vi "generate_plot.vi"(6 "High Voltage":sgl=2.0, 7 "Sens":dbl=12100000000000.0, 8 "error in":errorcluster, 10 "Vnoise":dbl=0.005, 11 "Dust Array":T2[](array[typedef])=[{"Dust Event ID"=59, "Integer Timestamp"=1340138392671, "Velocity"=19145.2, "Mass"=9.70909e-18, "Charge"=8.89689e-16, "Radius"=6.65219e-08, "Passed_3rd_Detector"=1, "High Voltage"=2.0, "+ High Voltage Supply"=0.0, "- High Voltage Supply"=0.0, "HV Control Difference"=0.0, "Vacuum Pressure"=0.0, "Radiation"=0.0, "Column Current"=0.0, "Lost Charge"=0.0, "Chain Current"=0.0, "Control High Voltage"=0.0, "Current Group Name:"="New Group Name", "Current Experiment Name:"="test", "Current Experiment Description:"="", "Estimate Source"=1, "Estimate Quality"=1.0, "File Location"=0, "Dust Type"="", "Dust Density"=0.0}, {"Dust Event ID"=61, "Integer Timestamp"=1340138406852, "Velocity"=9417.32, "Mass"=5.30434e-17, "Charge"=1.17605e-15, "Radius"=1.17161e-07, "Passed_3rd_Detector"=1, "High Voltage"=2.0, "+ High Voltage Supply"=0.0, "- High Voltage Supply"=0.0, "HV Control Difference"=0.0, "Vacuum Pressure"=0.0, "Radiation"=0.0, "Column Current"=0.0, "Lost Charge"=0.0, "Chain Current"=0.0, "Control High Voltage"=0.0, "Current Group Name:"="New Group Name", "Current Experiment Name:"="test", "Current Experiment Description:"="", "Estimate Source"=1, "Estimate Quality"=1.0, "File Location"=0, "Dust Type"="", "Dust Density"=0.0}, {"Dust Event ID"=63, "Integer Timestamp"=1340138434737, "Velocity"=6076.07, "Mass"=5.56419e-17, "Charge"=5.13556e-16, "Radius"=1.19044e-07, "Passed_3rd_Detector"=1, "High Voltage"=2.0, "+ High Voltage Supply"=0.0, "- High Voltage Supply"=0.0, "HV Control Difference"=0.0, "Vacuum Pressure"=0.0, "Radiation"=0.0, "Column Current"=0.0, "Lost Charge"=0.0, "Chain Current"=0.0, "Control High Voltage"=0.0, "Current Group Name:"="New Group Name", "Current Experiment Name:"="test", "Current Experiment Description:"="", "Estimate Source"=1, "Estimate Quality"=1.0, "File Location"=0, "Dust Type"="", "Dust Density"=0.0}, {"Dust Event ID"=65, "Integer Timestamp"=1340138517545, "Velocity"=5796.47, "Mass"=7.82766e-16, "Charge"=6.57505e-15, "Radius"=2.87375e-07, "Passed_3rd_Detector"=1, "High Voltage"=2.0, "+ High Voltage Supply"=0.0, "- High Voltage Supply"=0.0, "HV Control Difference"=0.0, "Vacuum Pressure"=0.0, "Radiation"=0.0, "Column Current"=0.0, "Lost Charge"=0.0, "Chain Current"=0.0, "Control High Voltage"=0.0, "Current Group Name:"="New Group Name", "Current Experiment Name:"="test", "Current Experiment Description:"="", "Estimate Source"=1, "Estimate Quality"=1.0, "File Location"=0, "Dust Type"="", "Dust Density"=0.0}, {"Dust Event ID"=66, "Integer Timestamp"=1340138518480, "Velocity"=9192.06, "Mass"=9.8916e-17, "Charge"=2.08945e-15, "Radius"=1.4421e-07, "Passed_3rd_Detector"=1, "High Voltage"=2.0, "+ High Voltage Supply"=0.0, "- High Voltage Supply"=0.0, "HV Control Difference"=0.0, "Vacuum Pressure"=0.0, "Radiation"=0.0, "Column Current"=0.0, "Lost Charge"=0.0, "Chain Current"=0.0, "Control High Voltage"=0.0, "Current Group Name:"="New Group Name", "Current Experiment Name:"="test", "Current Experiment Description:"="", "Estimate Source"=1, "Estimate Quality"=1.0, "File Location"=0, "Dust Type"="", "Dust Density"=0.0}, {"Dust Event ID"=67, "Integer Timestamp"=1340138532228, "Velocity"=34719.3, "Mass"=2.63602e-18, "Charge"=7.94385e-16, "Radius"=4.30746e-08, "Passed_3rd_Detector"=1, "High Voltage"=2.0, "+ High Voltage Supply"=0.0, "- High Voltage Supply"=0.0, "HV Control Difference"=0.0, "Vacuum Pressure"=0.0, "Radiation"=0.0, "Column Current"=0.0, "Lost Charge"=0.0, "Chain Current"=0.0, "Control High Voltage"=0.0, "Current Group Name:"="New Group Name", "Current Experiment Name:"="test", "Current Experiment Description:"="", "Estimate Source"=1, "Estimate Quality"=1.0, "File Location"=0, "Dust Type"="", "Dust Density"=0.0}, {"Dust Event ID"=68, "Integer Timestamp"=1340138545545, "Velocity"=7001.97, "Mass"=1.88556e-16, "Charge"=2.31111e-15, "Radius"=1.78807e-07, "Passed_3rd_Detector"=1, "High Voltage"=2.0, "+ High Voltage Supply"=0.0, "- High Voltage Supply"=0.0, "HV Control Difference"=0.0, "Vacuum Pressure"=0.0, "Radiation"=0.0, "Column Current"=0.0, "Lost Charge"=0.0, "Chain Current"=0.0, "Control High Voltage"=0.0, "Current Group Name:"="New Group Name", "Current Experiment Name:"="test", "Current Experiment Description:"="", "Estimate Source"=1, "Estimate Quality"=1.0, "File Location"=0, "Dust Type"="", "Dust Density"=0.0}, {"Dust Event ID"=73, "Integer Timestamp"=1340138752578, "Velocity"=19658.5, "Mass"=9.03687e-18, "Charge"=8.7309e-16, "Radius"=6.49498e-08, "Passed_3rd_Detector"=1, "High Voltage"=2.0, "+ High Voltage Supply"=0.0, "- High Voltage Supply"=0.0, "HV Control Difference"=0.0, "Vacuum Pressure"=0.0, "Radiation"=0.0, "Column Current"=0.0, "Lost Charge"=0.0, "Chain Current"=0.0, "Control High Voltage"=0.0, "Current Group Name:"="New Group Name", "Current Experiment Name:"="test", "Current Experiment Description:"="", "Estimate Source"=1, "Estimate Quality"=1.0, "File Location"=0, "Dust Type"="", "Dust Density"=0.0}, {"Dust Event ID"=74, "Integer Timestamp"=1340138757697, "Velocity"=26103.7, "Mass"=5.47988e-18, "Charge"=9.33502e-16, "Radius"=5.49746e-08, "Passed_3rd_Detector"=1, "High Voltage"=2.0, "+ High Voltage Supply"=0.0, "- High Voltage Supply"=0.0, "HV Control Difference"=0.0, "Vacuum Pressure"=0.0, "Radiation"=0.0, "Column Current"=0.0, "Lost Charge"=0.0, "Chain Current"=0.0, "Control High Voltage"=0.0, "Current Group Name:"="New Group Name", "Current Experiment Name:"="test", "Current Experiment Description:"="", "Estimate Source"=1, "Estimate Quality"=1.0, "File Location"=0, "Dust Type"="", "Dust Density"=0.0}, {"Dust Event ID"=75, "Integer Timestamp"=1340138762289, "Velocity"=11104.6, "Mass"=3.49915e-17, "Charge"=1.07872e-15, "Radius"=1.0199e-07, "Passed_3rd_Detector"=1, "High Voltage"=2.0, "+ High Voltage Supply"=0.0, "- High Voltage Supply"=0.0, "HV Control Difference"=0.0, "Vacuum Pressure"=0.0, "Radiation"=0.0, "Column Current"=0.0, "Lost Charge"=0.0, "Chain Current"=0.0, "Control High Voltage"=0.0, "Current Group Name:"="New Group Name", "Current Experiment Name:"="test", "Current Experiment Description:"="", "Estimate Source"=1, "Estimate Quality"=1.0, "File Location"=0, "Dust Type"="", "Dust Density"=0.0}, {"Dust Event ID"=76, "Integer Timestamp"=1340138792956, "Velocity"=7613.76, "Mass"=1.79901e-16, "Charge"=2.60719e-15, "Radius"=1.76029e-07, "Passed_3rd_Detector"=1, "High Voltage"=2.0, "+ High Voltage Supply"=0.0, "- High Voltage Supply"=0.0, "HV Control Difference"=0.0, "Vacuum Pressure"=0.0, "Radiation"=0.0, "Column Current"=0.0, "Lost Charge"=0.0, "Chain Current"=0.0, "Control High Voltage"=0.0, "Current Group Name:"="New Group Name", "Current Experiment Name:"="test", "Current Experiment Description:"="", "Estimate Source"=1, "Estimate Quality"=1.0, "File Location"=0, "Dust Type"="", "Dust Density"=0.0}, {"Dust Event ID"=80, "Integer Timestamp"=1340139107484, "Velocity"=34660.0, "Mass"=2.92065e-18, "Charge"=8.77155e-16, "Radius"=4.45723e-08, "Passed_3rd_Detector"=1, "High Voltage"=2.0, "+ High Voltage Supply"=0.0, "- High Voltage Supply"=0.0, "HV Control Difference"=0.0, "Vacuum Pressure"=0.0, "Radiation"=0.0, "Column Current"=0.0, "Lost Charge"=0.0, "Chain Current"=0.0, "Control High Voltage"=0.0, "Current Group Name:"="New Group Name", "Current Experiment Name:"="test", "Current Experiment Description:"="", "Estimate Source"=1, "Estimate Quality"=1.0, "File Location"=0, "Dust Type"="", "Dust Density"=0.0}, {"Dust Event ID"=85, "Integer Timestamp"=1340139269076, "Velocity"=7758.72, "Mass"=1.26144e-16, "Charge"=1.89839e-15, "Radius"=1.56385e-07, "Passed_3rd_Detector"=1, "High Voltage"=2.0, "+ High Voltage Supply"=0.0, "- High Voltage Supply"=0.0, "HV Control Difference"=0.0, "Vacuum Pressure"=0.0, "Radiation"=0.0, "Column Current"=0.0, "Lost Charge"=0.0, "Chain Current"=0.0, "Control High Voltage"=0.0, "Current Group Name:"="New Group Name", "Current Experiment Name:"="test", "Current Experiment Description:"="", "Estimate Source"=1, "Estimate Quality"=1.0, "File Location"=0, "Dust Type"="", "Dust Density"=0.0}, {"Dust Event ID"=90, "Integer Timestamp"=1340139421851, "Velocity"=7551.02, "Mass"=1.73571e-16, "Charge"=2.47417e-15, "Radius"=1.73939e-07, "Passed_3rd_Detector"=1, "High Voltage"=2.0, "+ High Voltage Supply"=0.0, "- High Voltage Supply"=0.0, "HV Control Difference"=0.0, "Vacuum Pressure"=0.0, "Radiation"=0.0, "Column Current"=0.0, "Lost Charge"=0.0, "Chain Current"=0.0, "Control High Voltage"=0.0, "Current Group Name:"="New Group Name", "Current Experiment Name:"="test", "Current Experiment Description:"="", "Estimate Source"=1, "Estimate Quality"=1.0, "File Location"=0, "Dust Type"="", "Dust Density"=0.0}, {"Dust Event ID"=92, "Integer Timestamp"=1340139600351, "Velocity"=17512.5, "Mass"=1.03329e-17, "Charge"=7.9224e-16, "Radius"=6.7917e-08, "Passed_3rd_Detector"=1, "High Voltage"=2.0, "+ High Voltage Supply"=0.0, "- High Voltage Supply"=0.0, "HV Control Difference"=0.0, "Vacuum Pressure"=0.0, "Radiation"=0.0, "Column Current"=0.0, "Lost Charge"=0.0, "Chain Current"=0.0, "Control High Voltage"=0.0, "Current Group Name:"="New Group Name", "Current Experiment Name:"="test", "Current Experiment Description:"="", "Estimate Source"=1, "Estimate Quality"=1.0, "File Location"=0, "Dust Type"="", "Dust Density"=0.0}, {"Dust Event ID"=95, "Integer Timestamp"=1340139724238, "Velocity"=28180.7, "Mass"=4.07113e-18, "Charge"=8.08274e-16, "Radius"=4.97902e-08, "Passed_3rd_Detector"=1, "High Voltage"=2.0, "+ High Voltage Supply"=0.0, "- High Voltage Supply"=0.0, "HV Control Difference"=0.0, "Vacuum Pressure"=0.0, "Radiation"=0.0, "Column Current"=0.0, "Lost Charge"=0.0, "Chain Current"=0.0, "Control High Voltage"=0.0, "Current Group Name:"="New Group Name", "Current Experiment Name:"="test", "Current Experiment Description:"="", "Estimate Source"=1, "Estimate Quality"=1.0, "File Location"=0, "Dust Type"="", "Dust Density"=0.0}, {"Dust Event ID"=97, "Integer Timestamp"=1340139740652, "Velocity"=7861.96, "Mass"=5.1459e-17, "Charge"=7.95176e-16, "Radius"=1.15983e-07, "Passed_3rd_Detector"=1, "High Voltage"=2.0, "+ High Voltage Supply"=0.0, "- High Voltage Supply"=0.0, "HV Control Difference"=0.0, "Vacuum Pressure"=0.0, "Radiation"=0.0, "Column Current"=0.0, "Lost Charge"=0.0, "Chain Current"=0.0, "Control High Voltage"=0.0, "Current Group Name:"="New Group Name", "Current Experiment Name:"="test", "Current Experiment Description:"="", "Estimate Source"=1, "Estimate Quality"=1.0, "File Location"=0, "Dust Type"="", "Dust Density"=0.0}, {"Dust Event ID"=105, "Integer Timestamp"=1340140151192, "Velocity"=6723.72, "Mass"=2.71295e-16, "Charge"=3.0662e-15, "Radius"=2.01861e-07, "Passed_3rd_Detector"=1, "High Voltage"=2.0, "+ High Voltage Supply"=0.0, "- High Voltage Supply"=0.0, "HV Control Difference"=0.0, "Vacuum Pressure"=0.0, "Radiation"=0.0, "Column Current"=0.0, "Lost Charge"=0.0, "Chain Current"=0.0, "Control High Voltage"=0.0, "Current Group Name:"="New Group Name", "Current Experiment Name:"="test", "Current Experiment Description:"="", "Estimate Source"=1, "Estimate Quality"=1.0, "File Location"=0, "Dust Type"="", "Dust Density"=0.0}, {"Dust Event ID"=108, "Integer Timestamp"=1340140254486, "Velocity"=42754.2, "Mass"=1.99038e-18, "Charge"=9.09563e-16, "Radius"=3.92239e-08, "Passed_3rd_Detector"=1, "High Voltage"=2.0, "+ High Voltage Supply"=0.0, "- High Voltage Supply"=0.0, "HV Control Difference"=0.0, "Vacuum Pressure"=0.0, "Radiation"=0.0, "Column Current"=0.0, "Lost Charge"=0.0, "Chain Current"=0.0, "Control High Voltage"=0.0, "Current Group Name:"="New Group Name", "Current Experiment Name:"="test", "Current Experiment Description:"="", "Estimate Source"=1, "Estimate Quality"=1.0, "File Location"=0, "Dust Type"="", "Dust Density"=0.0}, {"Dust Event ID"=111, "Integer Timestamp"=1340140356251, "Velocity"=16529.6, "Mass"=1.07981e-17, "Charge"=7.37587e-16, "Radius"=6.89215e-08, "Passed_3rd_Detector"=1, "High Voltage"=2.0, "+ High Voltage Supply"=0.0, "- High Voltage Supply"=0.0, "HV Control Difference"=0.0, "Vacuum Pressure"=0.0, "Radiation"=0.0, "Column Current"=0.0, "Lost Charge"=0.0, "Chain Current"=0.0, "Control High Voltage"=0.0, "Current Group Name:"="New Group Name", "Current Experiment Name:"="test", "Current Experiment Description:"="", "Estimate Source"=1, "Estimate Quality"=1.0, "File Location"=0, "Dust Type"="", "Dust Density"=0.0}, {"Dust Event ID"=112, "Integer Timestamp"=1340140385957, "Velocity"=8983.15, "Mass"=9.7223e-17, "Charge"=1.9614e-15, "Radius"=1.43382e-07, "Passed_3rd_Detector"=1, "High Voltage"=2.0, "+ High Voltage Supply"=0.0, "- High Voltage Supply"=0.0, "HV Control Difference"=0.0, "Vacuum Pressure"=0.0, "Radiation"=0.0, "Column Current"=0.0, "Lost Charge"=0.0, "Chain Current"=0.0, "Control High Voltage"=0.0, "Current Group Name:"="New Group Name", "Current Experiment Name:"="test", "Current Experiment Description:"="", "Estimate Source"=1, "Estimate Quality"=1.0, "File Location"=0, "Dust Type"="", "Dust Density"=0.0}, {"Dust Event ID"=113, "Integer Timestamp"=1340140387844, "Velocity"=29681.2, "Mass"=7.01615e-17, "Charge"=1.54526e-14, "Radius"=1.28609e-07, "Passed_3rd_Detector"=1, "High Voltage"=2.0, "+ High Voltage Supply"=0.0, "- High Voltage Supply"=0.0, "HV Control Difference"=0.0, "Vacuum Pressure"=0.0, "Radiation"=0.0, "Column Current"=0.0, "Lost Charge"=0.0, "Chain Current"=0.0, "Control High Voltage"=0.0, "Current Group Name:"="New Group Name", "Current Experiment Name:"="test", "Current Experiment Description:"="", "Estimate Source"=1, "Estimate Quality"=1.0, "File Location"=0, "Dust Type"="", "Dust Density"=0.0}, {"Dust Event ID"=116, "Integer Timestamp"=1340140419545, "Velocity"=30761.2, "Mass"=4.62537e-18, "Charge"=1.09419e-15, "Radius"=5.19542e-08, "Passed_3rd_Detector"=1, "High Voltage"=2.0, "+ High Voltage Supply"=0.0, "- High Voltage Supply"=0.0, "HV Control Difference"=0.0, "Vacuum Pressure"=0.0, "Radiation"=0.0, "Column Current"=0.0, "Lost Charge"=0.0, "Chain Current"=0.0, "Control High Voltage"=0.0, "Current Group Name:"="New Group Name", "Current Experiment Name:"="test", "Current Experiment Description:"="", "Estimate Source"=1, "Estimate Quality"=1.0, "File Location"=0, "Dust Type"="", "Dust Density"=0.0}, {"Dust Event ID"=118, "Integer Timestamp"=1340140449958, "Velocity"=23403.8, "Mass"=6.63985e-18, "Charge"=9.09224e-16, "Radius"=5.86082e-08, "Passed_3rd_Detector"=1, "High Voltage"=2.0, "+ High Voltage Supply"=0.0, "- High Voltage Supply"=0.0, "HV Control Difference"=0.0, "Vacuum Pressure"=0.0, "Radiation"=0.0, "Column Current"=0.0, "Lost Charge"=0.0, "Chain Current"=0.0, "Control High Voltage"=0.0, "Current Group Name:"="New Group Name", "Current Experiment Name:"="test", "Current Experiment Description:"="", "Estimate Source"=1, "Estimate Quality"=1.0, "File Location"=0, "Dust Type"="", "Dust Density"=0.0}] {"File Location" items=["Unknown"=-1, "Processing"=0, "Storage"=1]; "Estimate Source" items=["Any Source."=-2, "No Shot"=-1, "Basic Labview Estimate"=0, "IDL Estimate From Andrew"=1, "IDL Estimate From Tobin"=2, "Old Metadata"=3]}) -> (0 "error out":errorcluster, 3 "Dust Distribution":T1)   [LabVIEW 2013]
uses:
  Public API/Query_Dust_Event.ctl
  Controls/Estimate_source.ctl
  Controls/File_location.ctl
  Controls/Graph.ctl
panel:
  # "Dust Event"
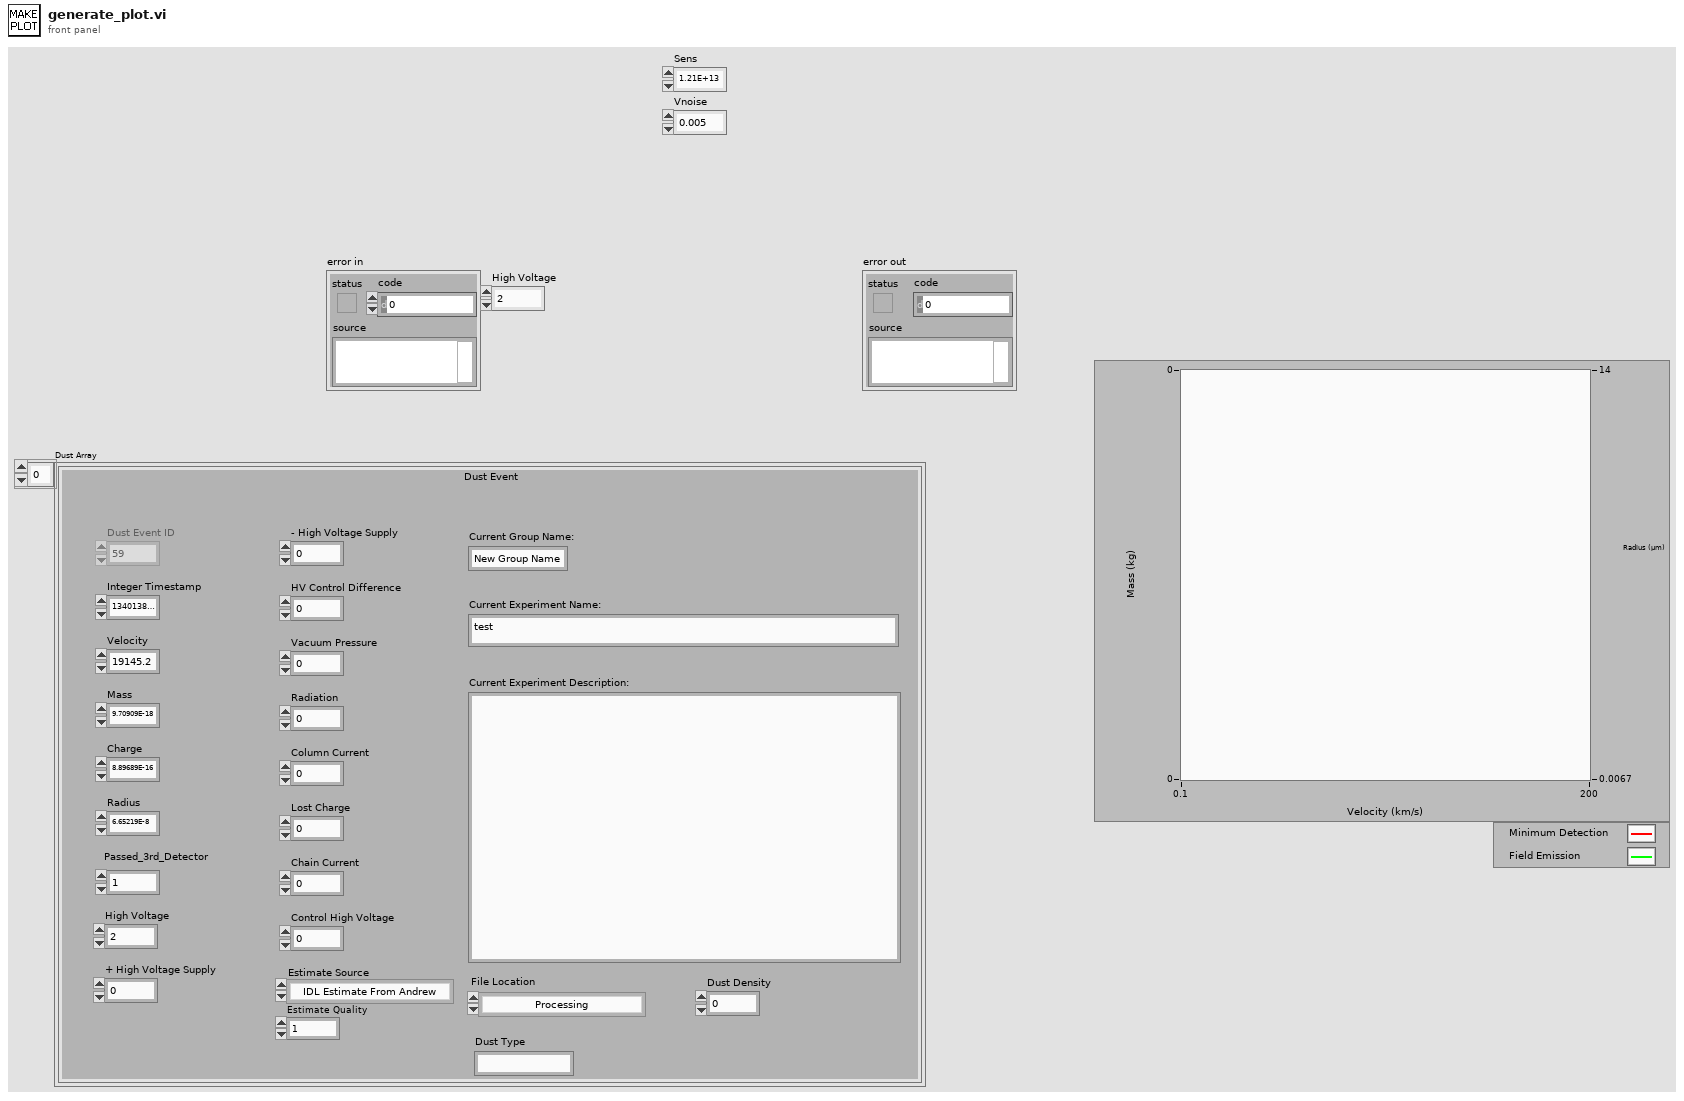
[diagram p1: front panel]
types:
  T1 = typedef "Graph.ctl" = cluster{cluster{"Vnoise":dbl, "Vnoise":dbl}[]}[]
  T2 = typedef "Query_Dust_Event.ctl" = cluster{"Dust Event ID":i64, "Integer Timestamp":i64, "Velocity":sgl, "Mass":sgl, "Charge":sgl, "Radius":sgl, "Passed_3rd_Detector":i8, "High Voltage":sgl, "+ High Voltage Supply":sgl, "- High Voltage Supply":sgl, "HV Control Difference":sgl, "Vacuum Pressure":sgl, "Radiation":sgl, "Column Current":sgl, "Lost Charge":sgl, "Chain Current":sgl, "Control High Voltage":sgl, "Current Group Name:":string, "Current Experiment Name:":string, "Current Experiment Description:":string, "Estimate Source":T3, "Estimate Quality":sgl, "File Location":T4, "Dust Type":string, "Dust Density":sgl}
  T3 = typedef "Estimate_source.ctl" = i8
  T4 = typedef "File_location.ctl" = i8
  T5 = cluster{cluster{"Vnoise":dbl, "Field Emission":dbl}[]}[]
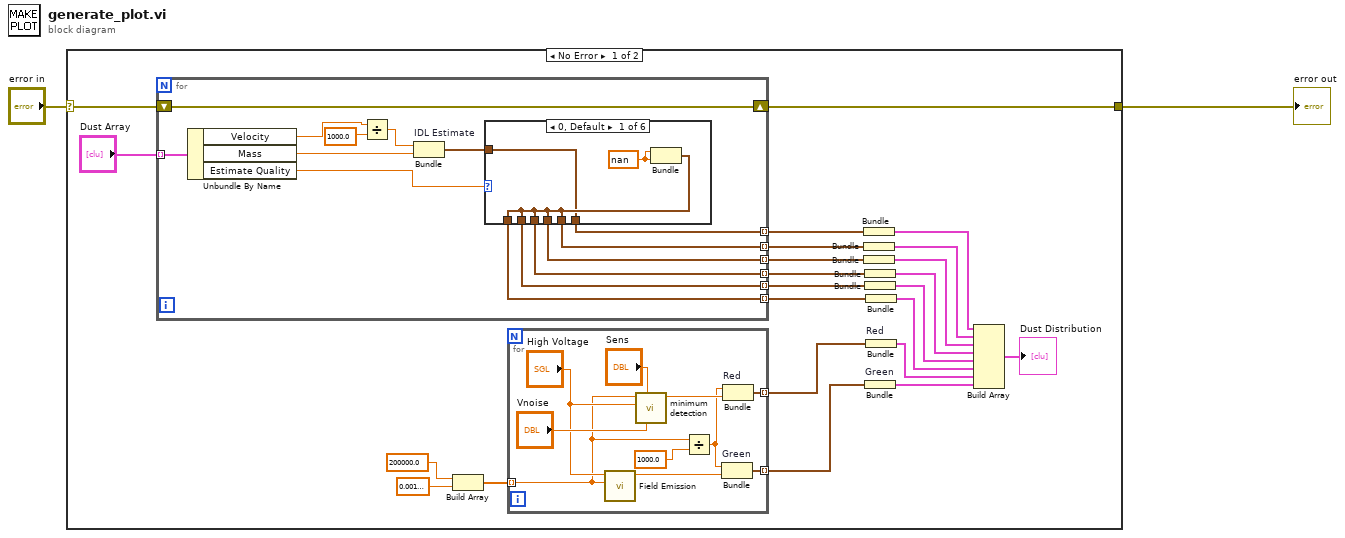
[diagram p0: block diagram]
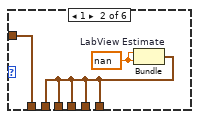
[diagram p2: hidden frame]
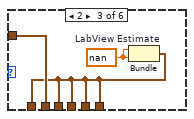
[diagram p3: hidden frame]
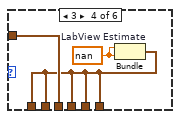
[diagram p4: hidden frame]
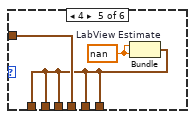
[diagram p5: hidden frame]
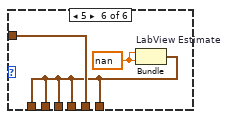
[diagram p6: hidden frame]
diagram:
  n1 = case shown="No Error" "error in" {
    selector: "error in" -> [w20 w68]
    tunnel: [w19 w68] -> w1
    frame No Error {
      n2 = for {
        tunnel: "Dust Array" -> [w47] mode=indexing
        tunnel: [w49] -> w25 mode=indexing
        shift-right: [w48] -> w19
        shift-left: w20 -> [w48]
        tunnel: [w41] -> w14 mode=indexing
        tunnel: [w40] -> w13 mode=indexing
        tunnel: [w39] -> w11 mode=indexing
        tunnel: [w38] -> w9 mode=indexing
        tunnel: [w36] -> w3 mode=indexing
        n3 = Unbundle By Name(w47) -> ("Velocity"=w46:sgl, "Mass"=w44:sgl, "Estimate Quality"=w42:sgl)
        n4 = Divide(x=w46, y=sgl 1000.0) -> (x/y=w43:sgl)
        n5 = Bundle "IDL Estimate"(w43, "Mass"=w44) -> (w37:cluster{sgl, "Mass":sgl})  [unwired: 1 in]
        n6 = case shown="0, Default" w42 {
          tunnel: [w51 w54 w56 w59 w62 w65] -> w49
          tunnel: w37 -> [w50 w54 w57 w61 w63 w66]
          tunnel: [w51 w53 w57 w59 w62 w65] -> w41
          tunnel: [w51 w53 w56 w61 w62 w65] -> w40
          tunnel: [w51 w53 w56 w59 w63 w65] -> w39
          tunnel: [w51 w53 w56 w59 w62 w66] -> w38
          tunnel: [w50 w53 w56 w59 w62 w65] -> w36
          frame 0, Default {
            w52 = nan ("Vnoise")
            n7 = Bundle ("LabView Estimate")("Vnoise"=w52, "Vnoise"=w52) -> (w51:cluster{"Vnoise":dbl, "Vnoise":dbl})  [unwired: 1 in]
          }
          frame 1 {
            w55 = nan ("Vnoise")
            n8 = Bundle "LabView Estimate"("Vnoise"=w55, "Vnoise"=w55) -> (w53:cluster{"Vnoise":dbl, "Vnoise":dbl})  [unwired: 1 in]
          }
          frame 2 {
            w58 = nan ("Vnoise")
            n9 = Bundle "LabView Estimate"("Vnoise"=w58, "Vnoise"=w58) -> (w56:cluster{"Vnoise":dbl, "Vnoise":dbl})  [unwired: 1 in]
          }
          frame 3 {
            w60 = nan ("Vnoise")
            n10 = Bundle "LabView Estimate"("Vnoise"=w60, "Vnoise"=w60) -> (w59:cluster{"Vnoise":dbl, "Vnoise":dbl})  [unwired: 1 in]
          }
          frame 4 {
            w64 = nan ("Vnoise")
            n11 = Bundle "LabView Estimate"("Vnoise"=w64, "Vnoise"=w64) -> (w62:cluster{"Vnoise":dbl, "Vnoise":dbl})  [unwired: 1 in]
          }
          frame 5 {
            w67 = nan ("Vnoise")
            n12 = Bundle "LabView Estimate"("Vnoise"=w67, "Vnoise"=w67) -> (w65:cluster{"Vnoise":dbl, "Vnoise":dbl})  [unwired: 1 in]
          }
        }
      }
      n13 = Build Array(sgl 200000.0 ("min value"), sgl 0.001 ("min value")) -> (w6:sgl[])
      n14 = for {
        tunnel: [w33] -> w22 mode=indexing
        tunnel: [w32] -> w21 mode=indexing
        tunnel: w6 -> [w27] mode=indexing
        n15 = call "Field Emission.vi"("Velocity"=w27, "Pelletron Volts"="High Voltage") -> ("Field Emission"=w31:dbl)  [unwired: 9 in]
        n16 = call "minimum detection.vi"("Sens"="Sens", "Vnoise"="Vnoise", "Pelletron Volts"="High Voltage", "Velocity"=w27) -> ("Minimum Detection"=w30:dbl)  [unwired: 7 in]
        n17 = Divide(x=w27, y=sgl 1000.0) -> (x/y=w26:sgl)
        n18 = Bundle "Green"(w26, "Field Emission"=w31) -> (w32:cluster{sgl, "Field Emission":dbl})  [unwired: 1 in]
        n19 = Bundle "Red"(w26, "Minimum Detection"=w30) -> (w33:cluster{sgl, "Minimum Detection":dbl})  [unwired: 1 in]
      }
      n20 = Bundle ("Scatter Plot")(w3) -> (w5:cluster{cluster{"Vnoise":dbl, "Vnoise":dbl}[]})  [unwired: 1 in]
      n21 = Bundle ("Scatter Plot")(w9) -> (w4:cluster{cluster{"Vnoise":dbl, "Vnoise":dbl}[]})  [unwired: 1 in]
      n22 = Bundle ("Scatter Plot")(w11) -> (w10:cluster{cluster{"Vnoise":dbl, "Vnoise":dbl}[]})  [unwired: 1 in]
      n23 = Bundle ("Scatter Plot")(w13) -> (w12:cluster{cluster{"Vnoise":dbl, "Vnoise":dbl}[]})  [unwired: 1 in]
      n24 = Bundle ("Scatter Plot")(w14) -> (w15:cluster{cluster{"Vnoise":dbl, "Vnoise":dbl}[]})  [unwired: 1 in]
      n25 = Bundle "Green"(w21) -> (w24:cluster{cluster{sgl, "Field Emission":dbl}[]})  [unwired: 1 in]
      n26 = Bundle ("Scatter Plot")(w25) -> (w16:cluster{cluster{"Vnoise":dbl, "Vnoise":dbl}[]})  [unwired: 1 in]
      n27 = Bundle "Red"(w22) -> (w23:cluster{cluster{sgl, "Minimum Detection":dbl}[]})  [unwired: 1 in]
      n28 = Build Array(w5, w4, w10, w12, w15, w16, w23, w24) -> (→"Dust Distribution":T5)
    }
    frame Error {
    }
  }
  "error out" <- w1
